vi "rsscope_core_global.vi"() -> ()   [LabVIEW 2018] (continued)
indicates the length of the data byte."}, {"Level"=4, "Class Only"=FALSE, "Identifier"="RSSCOPE_ATTR_CXPI_TRIGGER_DLC_CONDITION", "Descriptive Name"="CXPI Trigger DLC Condition", "Data Type"=0, "Command"="TRIG{Trigger}:CXPI:DLC:COND", "Access"=2, "Range Table"="rsscope_rngProtocolTriggerCondition", "Read Callback"="", "Write Callback"="", "Supported Models"="", "Instrument Options"="K76", "Flags"=0, "Help"="Set the condition for the DLC. You can define an exact value or a value range.\n\nAvailable Repeated Capabilities:\nTrigger: TrigA, TrigB, TrigR\r\n\nRemote-control command(s):\nTRIGger<m>:CXPI:DLC:CONDition"}, {"Level"=4, "Class Only"=FALSE, "Identifier"="RSSCOPE_ATTR_CXPI_TRIGGER_DLC_MIN", "Descriptive Name"="CXPI Trigger DLC Min", "Data Type"=2, "Command"="TRIG{Trigger}:CXPI:DLC:MIN", "Access"=2, "Range Table"="", "Read Callback"="", "Write Callback"="", "Supported Models"="", "Instrument Options"="K76", "Flags"=0, "Help"="Specifies a DLC pattern, or sets the start value of a pattern range.\n\nValid Values:\nBinary pattern string consisting of 1; 0; or X (any bit).\n\nAvailable Repeated Capabilities:\nTrigger: TrigA, TrigB, TrigR\r\n\nRemote-control command(s):\nTRIGger<m>:CXPI:DLC:MIN"}, {"Level"=4, "Class Only"=FALSE, "Identifier"="RSSCOPE_ATTR_CXPI_TRIGGER_DLC_MAX", "Descriptive Name"="CXPI Trigger DLC Max", "Data Type"=2, "Command"="TRIG{Trigger}:CXPI:DLC:MAX", "Access"=2, "Range Table"="", "Read Callback"="", "Write Callback"="", "Supported Models"="", "Instrument Options"="K76", "Flags"=0, "Help"="Sets the end value of a data type range for condition In Range or Out of Range. \n\nValid Values:\nBinary pattern string consisting of 1; 0; or X (any bit).\n\nAvailable Repeated Capabilities:\nTrigger: TrigA, TrigB, TrigR\r\n\nRemote-control command(s):\nTRIGger<m>:CXPI:DLC:MAX"}, {"Level"=3, "Class Only"=TRUE, "Identifier"="", "Descriptive Name"="DLC Extend", "Data Type"=0, "Command"="", "Access"=0, "Range Table"="", "Read Callback"="", "Write Callback"="", "Supported Models"="", "Instrument Options"="", "Flags"=0, "Help"="Sets the extension data length code, which indicates the length of the data byte of a long frame."}, {"Level"=4, "Class Only"=FALSE, "Identifier"="RSSCOPE_ATTR_CXPI_TRIGGER_DLC_EXTEND_CONDITION", "Descriptive Name"="CXPI Trigger DLC Extend Condition", "Data Type"=0, "Command"="TRIG{Trigger}:CXPI:DEXT:COND", "Access"=2, "Range Table"="rsscope_rngProtocolTriggerCondition", "Read Callback"="", "Write Callback"="", "Supported Models"="", "Instrument Options"="K76", "Flags"=0, "Help"="Set the condition for the DLC extend value. You can define an exact value or a value range.\n\nAvailable Repeated Capabilities:\nTrigger: TrigA, TrigB, TrigR\r\n\nRemote-control command(s):\nTRIGger<m>:CXPI:DEXTension:CONDition"}, {"Level"=4, "Class Only"=FALSE, "Identifier"="RSSCOPE_ATTR_CXPI_TRIGGER_DLC_EXTEND_MIN", "Descriptive Name"="CXPI Trigger DLC Extend Min", "Data Type"=2, "Command"="TRIG{Trigger}:CXPI:DEXT:MIN", "Access"=2, "Range Table"="", "Read Callback"="", "Write Callback"="", "Supported Models"="", "Instrument Options"="K76", "Flags"=0, "Help"="Specifies a data extension bit pattern, or sets the start value of a pattern range.\n\nValid Values:\nBinary pattern string consisting of 1; 0; or X (any bit).\n\nAvailable Repeated Capabilities:\nTrigger: TrigA, TrigB, TrigR\r\n\nRemote-control command(s):\nTRIGger<m>:CXPI:DEXTension:MIN"}, {"Level"=4, "Class Only"=FALSE, "Identifier"="RSSCOPE_ATTR_CXPI_TRIGGER_DLC_EXTEND_MAX", "Descriptive Name"="CXPI Trigger DLC Extend Max", "Data Type"=2, "Command"="TRIG{Trigger}:CXPI:DEXT:MAX", "Access"=2, "Range Table"="", "Read Callback"="", "Write Callback"="", "Supported Models"="", "Instrument Options"="K76", "Flags"=0, "Help"="Sets the end value of a DLC extend range for condition In Range or Out of Range. \n\nValid Values:\nBinary pattern string consisting of 1; 0; or X (any bit).\n\nAvailable Repeated Capabilities:\nTrigger: TrigA, TrigB, TrigR\r\n\nRemote-control command(s):\nTRIGger<m>:CXPI:DEXTension:MAX"}, {"Level"=3, "Class Only"=TRUE, "Identifier"="", "Descriptive Name"="Data", "Data Type"=0, "Command"="", "Access"=0, "Range Table"="", "Read Callback"="", "Write Callback"="", "Supported Models"="", "Instrument Options"="", "Flags"=0, "Help"="The data setup consists of the condition and one or two identifier pattern."}, {"Level"=4, "Class Only"=FALSE, "Identifier"="RSSCOPE_ATTR_CXPI_TRIGGER_DATA_CONDITION", "Descriptive Name"="CXPI Trigger Data Condition", "Data Type"=0, "Command"="TRIG{Trigger}:CXPI:DATA:DCON", "Access"=2, "Range Table"="rsscope_rngCXPIDataCondition", "Read Callback"="", "Write Callback"="", "Supported Models"="", "Instrument Options"="K76", "Flags"=0, "Help"="Sets the condition for the data pattern. You can define no value, an exact value or a value range.\n\nAvailable Repeated Capabilities:\nTrigger: TrigA, TrigB, TrigR\r\n\nRemote-control command(s):\nTRIGger<m>:CXPI:DATA:DCONdition"}, {"Level"=4, "Class Only"=FALSE, "Identifier"="RSSCOPE_ATTR_CXPI_TRIGGER_DATA_MIN", "Descriptive Name"="CXPI Trigger Data Min", "Data Type"=2, "Command"="TRIG{Trigger}:CXPI:DATA:DMIN", "Access"=2, "Range Table"="", "Read Callback"="", "Write Callback"="", "Supported Models"="", "Instrument Options"="K76", "Flags"=0, "Help"="Specifies a data bit pattern, or sets the start value of a pattern range.\n\nValid Values:\nBinary pattern string consisting of 1; 0; or X (any bit).\n\nAvailable Repeated Capabilities:\nTrigger: TrigA, TrigB, TrigR\r\n\nRemote-control command(s):\nTRIGger<m>:CXPI:DATA:DMIN"}, {"Level"=4, "Class Only"=FALSE, "Identifier"="RSSCOPE_ATTR_CXPI_TRIGGER_DATA_MAX", "Descriptive Name"="CXPI Trigger Data Max", "Data Type"=2, "Command"="TRIG{Trigger}:CXPI:DATA:DMAX", "Access"=2, "Range Table"="", "Read Callback"="", "Write Callback"="", "Supported Models"="", "Instrument Options"="K76", "Flags"=0, "Help"="Sets the end value of a data type range for condition In Range or Out of Range. \n\nValid Values:\nBinary pattern string consisting of 1; 0; or X (any bit).\n\nAvailable Repeated Capabilities:\nTrigger: TrigA, TrigB, TrigR\r\n\nRemote-control command(s):\nTRIGger<m>:CXPI:DATA:DMAX"}, {"Level"=3, "Class Only"=TRUE, "Identifier"="", "Descriptive Name"="Index", "Data Type"=0, "Command"="", "Access"=0, "Range Table"="", "Read Callback"="", "Write Callback"="", "Supported Models"="", "Instrument Options"="", "Flags"=0, "Help"="The data index setup consists of the condition and one or two index patterns."}, {"Level"=4, "Class Only"=FALSE, "Identifier"="RSSCOPE_ATTR_CXPI_TRIGGER_INDEX_CONDITION", "Descriptive Name"="CXPI Trigger Index Condition", "Data Type"=0, "Command"="TRIG{Trigger}:CXPI:DATA:ICON", "Access"=2, "Range Table"="rsscope_rngProtocolTriggerCondition", "Read Callback"="", "Write Callback"="", "Supported Models"="", "Instrument Options"="K76", "Flags"=0, "Help"="Set the condition for the data index value. You can define an exact value or a value range.\n\nAvailable Repeated Capabilities:\nTrigger: TrigA, TrigB, TrigR\r\n\nRemote-control command(s):\nTRIGger<m>:CXPI:DATA:ICONdition"}, {"Level"=4, "Class Only"=FALSE, "Identifier"="RSSCOPE_ATTR_CXPI_TRIGGER_INDEX_MIN", "Descriptive Name"="CXPI Trigger Index Min", "Data Type"=0, "Command"="TRIG{Trigger}:CXPI:DATA:IMIN", "Access"=2, "Range Table"="", "Read Callback"="", "Write Callback"="", "Supported Models"="", "Instrument Options"="K76", "Flags"=0, "Help"="Specifies a data index bit pattern, or sets the start value of a pattern range.\n\nAvailable Repeated Capabilities:\nTrigger: TrigA, TrigB, TrigR\r\n\nRemote-control command(s):\nTRIGger<m>:CXPI:DATA:IMIN"}, {"Level"=4, "Class Only"=FALSE, "Identifier"="RSSCOPE_ATTR_CXPI_TRIGGER_INDEX_MAX", "Descriptive Name"="CXPI Trigger Index Max", "Data Type"=0, "Command"="TRIG{Trigger}:CXPI:DATA:IMAX", "Access"=2, "Range Table"="", "Read Callback"="", "Write Callback"="", "Supported Models"="", "Instrument Options"="K76", "Flags"=0, "Help"="Sets the end value of a data index range for condition In Range or Out of Range.\n\nAvailable Repeated Capabilities:\nTrigger: TrigA, TrigB, TrigR\r\n\nRemote-control command(s):\nTRIGger<m>:CXPI:DATA:IMAX"}, {"Level"=3, "Class Only"=TRUE, "Identifier"="", "Descriptive Name"="Error", "Data Type"=0, "Command"="", "Access"=0, "Range Table"="", "Read Callback"="", "Write Callback"="", "Supported Models"="", "Instrument Options"="", "Flags"=0, "Help"="Trigger on selected error types."}, {"Level"=4, "Class Only"=FALSE, "Identifier"="RSSCOPE_ATTR_CXPI_TRIGGER_ERROR_CRC", "Descriptive Name"="CXPI Trigger Error CRC", "Data Type"=3, "Command"="TRIG{Trigger}:CXPI:ERR:CRC", "Access"=2, "Range Table"="", "Read Callback"="", "Write Callback"="", "Supported Models"="", "Instrument Options"="K76", "Flags"=0, "Help"="Triggers on a cyclic redundancy check error.\n\nAvailable Repeated Capabilities:\nTrigger: TrigA, TrigB, TrigR\r\n\nRemote-control command(s):\nTRIGger<m>:CXPI:ERRor:CRC"}, {"Level"=4, "Class Only"=FALSE, "Identifier"="RSSCOPE_ATTR_CXPI_TRIGGER_ERROR_DLC", "Descriptive Name"="CXPI Trigger Error DLC", "Data Type"=3, "Command"="TRIG{Trigger}:CXPI:ERR:DLC", "Access"=2, "Range Table"="", "Read Callback"="", "Write Callback"="", "Supported Models"="", "Instrument Options"="K76", "Flags"=0, "Help"="Triggers on a data length code (DLC) error.\n\nAvailable Repeated Capabilities:\nTrigger: TrigA, TrigB, TrigR\r\n\nRemote-control command(s):\nTRIGger<m>:CXPI:ERRor:DLC"}, {"Level"=4, "Class Only"=FALSE, "Identifier"="RSSCOPE_ATTR_CXPI_TRIGGER_ERROR_IBS", "Descriptive Name"="CXPI Trigger Error IBS", "Data Type"=3, "Command"="TRIG{Trigger}:CXPI:ERR:IBS", "Access"=2, "Range Table"="", "Read Callback"="", "Write Callback"="", "Supported Models"="", "Instrument Options"="K76", "Flags"=0, "Help"="Triggers on an inter-byte-space (IBS) error.\n\nAvailable Repeated Capabilities:\nTrigger: TrigA, TrigB, TrigR\r\n\nRemote-control command(s):\nTRIGger<m>:CXPI:ERRor:IBS"}, {"Level"=4, "Class Only"=FALSE, "Identifier"="RSSCOPE_ATTR_CXPI_TRIGGER_ERROR_IFS", "Descriptive Name"="CXPI Trigger Error IFS", "Data Type"=3, "Command"="TRIG{Trigger}:CXPI:ERR:IFS", "Access"=2, "Range Table"="", "Read Callback"="", "Write Callback"="", "Supported Models"="", "Instrument Options"="K76", "Flags"=0, "Help"="Triggers on an inter-frame-space (IFS) error.\n\nAvailable Repeated Capabilities:\nTrigger: TrigA, TrigB, TrigR\r\n\nRemote-control command(s):\nTRIGger<m>:CXPI:ERRor:IFS"}, {"Level"=4, "Class Only"=FALSE, "Identifier"="RSSCOPE_ATTR_CXPI_TRIGGER_ERROR_LENGTH", "Descriptive Name"="CXPI Trigger Error Length", "Data Type"=3, "Command"="TRIG{Trigger}:CXPI:ERR:LENG", "Access"=2, "Range Table"="", "Read Callback"="", "Write Callback"="", "Supported Models"="", "Instrument Options"="K76", "Flags"=0, "Help"="Triggers on a length error.\n\nAvailable Repeated Capabilities:\nTrigger: TrigA, TrigB, TrigR\r\n\nRemote-control command(s):\nTRIGger<m>:CXPI:ERRor:LENGth"}, {"Level"=4, "Class Only"=FALSE, "Identifier"="RSSCOPE_ATTR_CXPI_TRIGGER_ERROR_PARITY", "Descriptive Name"="CXPI Trigger Error Parity", "Data Type"=3, "Command"="TRIG{Trigger}:CXPI:ERR:PAR", "Access"=2, "Range Table"="", "Read Callback"="", "Write Callback"="", "Supported Models"="", "Instrument Options"="K76", "Flags"=0, "Help"="Triggers on a parity error indicating a transmission error.\n\nAvailable Repeated Capabilities:\nTrigger: TrigA, TrigB, TrigR\r\n\nRemote-control command(s):\nTRIGger<m>:CXPI:ERRor:PARity"}, {"Level"=4, "Class Only"=FALSE, "Identifier"="RSSCOPE_ATTR_CXPI_TRIGGER_ERROR_UART", "Descriptive Name"="CXPI Trigger Error UART", "Data Type"=3, "Command"="TRIG{Trigger}:CXPI:ERR:UART", "Access"=2, "Range Table"="", "Read Callback"="", "Write Callback"="", "Supported Models"="", "Instrument Options"="K76", "Flags"=0, "Help"="Triggers on an UART error.\n\nAvailable Repeated Capabilities:\nTrigger: TrigA, TrigB, TrigR\r\n\nRemote-control command(s):\nTRIGger<m>:CXPI:ERRor:UART"}, {"Level"=2, "Class Only"=TRUE, "Identifier"="", "Descriptive Name"="PCIe", "Data Type"=0, "Command"="", "Access"=0, "Range Table"="", "Read Callback"="", "Write Callback"="", "Supported Models"="", "Instrument Options"="", "Flags"=0, "Help"="Configures PCIe trigger."}, {"Level"=3, "Class Only"=FALSE, "Identifier"="RSSCOPE_ATTR_PCIE_TRIGGER_TYPE", "Descriptive Name"="PCIe Trigger Type", "Data Type"=0, "Command"="TRIG{Trigger}:PCIE:TYPE", "Access"=2, "Range Table"="RsScope_rngPCIeTriggerType", "Read Callback"="", "Write Callback"="", "Supported Models"="RTO|RTP", "Instrument Options"="K72", "Flags"=0, "Help"="Sets the trigger type for the PCI express analysis.\n\nAvailable Repeated Capabilities:\nTrigger: TrigA, TrigB, TrigR\r\n\nRemote-control command(s):\nTRIGger<m>:PCIE:TYPE"}, {"Level"=3, "Class Only"=FALSE, "Identifier"="RSSCOPE_ATTR_PCIE_TRIGGER_LEVEL", "Descriptive Name"="PCIe Trigger Level", "Data Type"=1, "Command"="TRIG{Trigger}:PCIE:TRGL", "Access"=2, "Range Table"="RsScope_rngPCIeTriggerLevel", "Read Callback"="", "Write Callback"="", "Supported Models"="", "Instrument Options"="", "Flags"=0, "Help"="Sets the trigger level for PCIe Gen 3.\n\nAvailable Repeated Capabilities:\nTrigger: TrigA, TrigB, TrigR\r\n\nRemote-control command(s):\nTRIGger<m>:PCIE:TRGLevel"}, {"Level"=3, "Class Only"=TRUE, "Identifier"="", "Descriptive Name"="TLP", "Data Type"=0, "Command"="", "Access"=0, "Range Table"="", "Read Callback"="", "Write Callback"="", "Supported Models"="", "Instrument Options"="", "Flags"=0, "Help"="Triggers on a transaction type."}, {"Level"=4, "Class Only"=FALSE, "Identifier"="RSSCOPE_ATTR_PCIE_TRIGGER_TLP", "Descriptive Name"="PCIe Trigger TLP", "Data Type"=0, "Command"="TRIG{Trigger}:PCIE:TLP:TYPE", "Access"=2, "Range Table"="RsScope_rngPCIeTLP", "Read Callback"="", "Write Callback"="", "Supported Models"="RTO|RTP", "Instrument Options"="K72", "Flags"=0, "Help"="Sets the transaction type to be triggered on for the transaction layer type trigger.\n\nAvailable Repeated Capabilities:\nTrigger: TrigA, TrigB, TrigR\r\n\nRemote-control command(s):\nTRIGger<m>:PCIE:TLP:TYPE"}, {"Level"=4, "Class Only"=FALSE, "Identifier"="RSSCOPE_ATTR_PCIE_TRIGGER_TLP_SEQUENCE_NUMBER", "Descriptive Name"="PCIe Trigger TLP Sequence Number", "Data Type"=2, "Command"="TRIG{Trigger}:PCIE:TLP:SNUM", "Access"=2, "Range Table"="", "Read Callback"="", "Write Callback"="", "Supported Models"="RTO|RTP", "Instrument Options"="K72", "Flags"=0, "Help"="Sets the sequence number to be triggered on for the transaction layer type trigger.\n\nAvailable Repeated Capabilities:\nTrigger: TrigA, TrigB, TrigR\r\n\nRemote-control command(s):\nTRIGger<m>:PCIE:TLP:SNUM"}, {"Level"=4, "Class Only"=FALSE, "Identifier"="RSSCOPE_ATTR_PCIE_TRIGGER_TLP_TC", "Descriptive Name"="PCIe Trigger TLP TC", "Data Type"=0, "Command"="TRIG{Trigger}:PCIE:TLP:TCHN", "Access"=2, "Range Table"="RsScope_rngPCIeTLPTC", "Read Callback"="", "Write Callback"="", "Supported Models"="RTO|RTP", "Instrument Options"="K72", "Flags"=0, "Help"="Sets the traffic class to be triggered on for the transaction layer type trigger.\n\nAvailable Repeated Capabilities:\nTrigger: TrigA, TrigB, TrigR\r\n\nRemote-control command(s):\nTRIGger<m>:PCIE:TLP:TCHN"}, {"Level"=4, "Class Only"=FALSE, "Identifier"="RSSCOPE_ATTR_PCIE_TRIGGER_TLP_ORDERING", "Descriptive Name"="PCIe Trigger TLP Ordering", "Data Type"=0, "Command"="TRIG{Trigger}:PCIE:TLP:ORDE", "Access"=2, "Range Table"="RsScope_rngPCIeTLPOrdering", "Read Callback"="", "Write Callback"="", "Supported Models"="RTO|RTP", "Instrument Options"="K72", "Flags"=0, "Help"="Sets the ordering type to be triggered on for the transaction layer type trigger.\n\nAvailable Repeated Capabilities:\nTrigger: TrigA, TrigB, TrigR\r\n\nRemote-control command(s):\nTRIGger<m>:PCIE:TLP:ORDE"}, {"Level"=4, "Class Only"=FALSE, "Identifier"="RSSCOPE_ATTR_PCIE_TRIGGER_TLP_SNOOP", "Descriptive Name"="PCIe Trigger TLP Snoop", "Data Type"=0, "Command"="TRIG{Trigger}:PCIE:TLP:SNOO", "Access"=2, "Range Table"="RsScope_rngPCIeTLPSnoop", "Read Callback"="", "Write Callback"="", "Supported Models"="RTO|RTP", "Instrument Options"="K72", "Flags"=0, "Help"="Triggers on a snoop state.\n\nAvailable Repeated Capabilities:\nTrigger: TrigA, TrigB, TrigR\r\n\nRemote-control command(s):\nTRIGger<m>:PCIE:TLP:SNOO"}, {"Level"=4, "Class Only"=FALSE, "Identifier"="RSSCOPE_ATTR_PCIE_TRIGGER_TLP_REQUESTER_ID", "Descriptive Name"="PCIe Trigger TLP Requester ID", "Data Type"=2, "Command"="TRIG{Trigger}:PCIE:TLP:REID", "Access"=2, "Range Table"="", "Read Callback"="", "Write Callback"="", "Supported Models"="RTO|RTP", "Instrument Options"="K72", "Flags"=0, "Help"="Sets the requester ID to be triggered on for the transaction layer type trigger.\n\nAvailable Repeated Capabilities:\nTrigger: TrigA, TrigB, TrigR\r\n\nRemote-control command(s):\nTRIGger<m>:PCIE:TLP:REID"}, {"Level"=4, "Class Only"=FALSE, "Identifier"="RSSCOPE_ATTR_PCIE_TRIGGER_TLP_DEVICE_ID", "Descriptive Name"="PCIe Trigger TLP Device ID", "Data Type"=2, "Command"="TRIG{Trigger}:PCIE:TLP:DEID", "Access"=2, "Range Table"="", "Read Callback"="", "Write Callback"="", "Supported Models"="RTO|RTP", "Instrument Options"="K72", "Flags"=0, "Help"="Sets the device ID to be triggered on for the transaction layer type trigger.\n\nAvailable Repeated Capabilities:\nTrigger: TrigA, TrigB, TrigR\r\n\nRemote-control command(s):\nTRIGger<m>:PCIE:TLP:DEID"}, {"Level"=4, "Class Only"=FALSE, "Identifier"="RSSCOPE_ATTR_PCIE_TRIGGER_TLP_READ_WRITE", "Descriptive Name"="PCIe Trigger TLP Read Write", "Data Type"=0, "Command"="TRIG{Trigger}:PCIE:TLP:MERW", "Access"=2, "Range Table"="RsScope_rngPCIeTLPReadWrite", "Read Callback"="", "Write Callback"="", "Supported Models"="RTO|RTP", "Instrument Options"="K72", "Flags"=0, "Help"="Sets the read/ write type to be triggered on for the transaction layer type trigger.\n\nAvailable Repeated Capabilities:\nTrigger: TrigA, TrigB, TrigR\r\n\nRemote-control command(s):\nTRIGger<m>:PCIE:TLP:MERW"}, {"Level"=4, "Class Only"=FALSE, "Identifier"="RSSCOPE_ATTR_PCIE_TRIGGER_TLP_ADDRESS_TYPE", "Descriptive Name"="PCIe Trigger TLP Address Type", "Data Type"=0, "Command"="TRIG{Trigger}:PCIE:TLP:ADRT", "Access"=2, "Range Table"="RsScope_rngPCIeTLPAddressType", "Read Callback"="", "Write Callback"="", "Supported Models"="RTO|RTP", "Instrument Options"="K72", "Flags"=0, "Help"="Sets the address type to be triggered on for the transaction layer type trigger.\n\nAvailable Repeated Capabilities:\nTrigger: TrigA, TrigB, TrigR\r\n\nRemote-control command(s):\nTRIGger<m>:PCIE:TLP:ADRT"}, {"Level"=4, "Class Only"=FALSE, "Identifier"="RSSCOPE_ATTR_PCIE_TRIGGER_TLP_TYPE", "Descriptive Name"="PCIe Trigger TLP Type", "Data Type"=0, "Command"="TRIG{Trigger}:PCIE:TLP:CFGT", "Access"=2, "Range Table"="RsScope_rngPCIeTLPType", "Read Callback"="", "Write Callback"="", "Supported Models"="RTO|RTP", "Instrument Options"="K72", "Flags"=0, "Help"="Triggers on a configuration type.\n\nAvailable Repeated Capabilities:\nTrigger: TrigA, TrigB, TrigR\r\n\nRemote-control command(s):\nTRIGger<m>:PCIE:TLP:CFGT"}, {"Level"=4, "Class Only"=FALSE, "Identifier"="RSSCOPE_ATTR_PCIE_TRIGGER_TLP_AT_TYPE", "Descriptive Name"="PCIe Trigger TLP AT Type", "Data Type"=0, "Command"="TRIG{Trigger}:PCIE:TLP:AT", "Access"=2, "Range Table"="RsScope_rngTriggerTLPATType", "Read Callback"="", "Write Callback"="", "Supported Models"="", "Instrument Options"="", "Flags"=0, "Help"="Sets the AT Type.\n\nAvailable Repeated Capabilities:\nTrigger: TrigA, TrigB, TrigR\r\n\nRemote-control command(s):\nTRIGger<m>:PCIE:TLP:AT"}, {"Level"=4, "Class Only"=FALSE, "Identifier"="RSSCOPE_ATTR_PCIE_TRIGGER_TLP_ROUTING", "Descriptive Name"="PCIe Trigger TLP Routing", "Data Type"=0, "Command"="TRIG{Trigger}:PCIE:TLP:MSGR", "Access"=2, "Range Table"="RsScope_rngPCIeTLPRouting", "Read Callback"="", "Write Callback"="", "Supported Models"="RTO|RTP", "Instrument Options"="K72", "Flags"=0, "Help"="Sets the message routing type to be triggered on for the transaction layer type trigger.\n\nAvailable Repeated Capabilities:\nTrigger: TrigA, TrigB, TrigR\r\n\nRemote-control command(s):\nTRIGger<m>:PCIE:TLP:MSGR"}, {"Level"=4, "Class Only"=FALSE, "Identifier"="RSSCOPE_ATTR_PCIE_TRIGGER_TLP_MESSAGE_CODE", "Descriptive Name"="PCIe Trigger TLP Message Code", "Data Type"=2, "Command"="TRIG{Trigger}:PCIE:TLP:MSGC", "Access"=2, "Range Table"="", "Read Callback"="", "Write Callback"="", "Supported Models"="RTO|RTP", "Instrument Options"="K72", "Flags"=0, "Help"="Sets the message code to be triggered on for the transaction layer type trigger.\n\nAvailable Repeated Capabilities:\nTrigger: TrigA, TrigB, TrigR\r\n\nRemote-control command(s):\nTRIGger<m>:PCIE:TLP:MSGC"}, {"Level"=4, "Class Only"=FALSE, "Identifier"="RSSCOPE_ATTR_PCIE_TRIGGER_TLP_STATUS", "Descriptive Name"="PCIe Trigger TLP Status", "Data Type"=0, "Command"="TRIG{Trigger}:PCIE:TLP:CPLS", "Access"=2, "Range Table"="RsScope_rngPCIeTLPStatus", "Read Callback"="", "Write Callback"="", "Supported Models"="RTO|RTP", "Instrument Options"="K72", "Flags"=0, "Help"="Sets the completion status to be triggered on for the transaction layer type trigger.\n\nAvailable Repeated Capabilities:\nTrigger: TrigA, TrigB, TrigR\r\n\nRemote-control command(s):\nTRIGger<m>:PCIE:TLP:CPLS"}, {"Level"=4, "Class Only"=FALSE, "Identifier"="RSSCOPE_ATTR_PCIE_TRIGGER_TLP_COMPLETER_ID", "Descriptive Name"="PCIe Trigger TLP Completer ID", "Data Type"=2, "Command"="TRIG{Trigger}:PCIE:TLP:CPID", "Access"=2, "Range Table"="", "Read Callback"="", "Write Callback"="", "Supported Models"="RTO|RTP", "Instrument Options"="K72", "Flags"=0, "Help"="Sets the completer ID to be triggered on for the transaction layer type trigger.\n\nAvailable Repeated Capabilities:\nTrigger: TrigA, TrigB, TrigR\r\n\nRemote-control command(s):\nTRIGger<m>:PCIE:TLP:CPID"}, {"Level"=3, "Class Only"=TRUE, "Identifier"="", "Descriptive Name"="DLLP", "Data Type"=0, "Command"="", "Access"=0, "Range Table"="", "Read Callback"="", "Write Callback"="", "Supported Models"="", "Instrument Options"="", "Flags"=0, "Help"="Configures data link layer trigger."}, {"Level"=4, "Class Only"=FALSE, "Identifier"="RSSCOPE_ATTR_PCIE_TRIGGER_DLLP", "Descriptive Name"="PCIe Trigger DLLP", "Data Type"=0, "Command"="TRIG{Trigger}:PCIE:DLLP:TYPE", "Access"=2, "Range Table"="RsScope_rngPCIeDLLP", "Read Callback"="", "Write Callback"="", "Supported Models"="RTO|RTP", "Instrument Options"="K72", "Flags"=0, "Help"="Sets the DLLP t type to be triggered on for the data link layer trigger.\n\nAvailable Repeated Capabilities:\nTrigger: TrigA, TrigB, TrigR\r\n\nRemote-control command(s):\nTRIGger<m>:PCIE:DLLP:TYPE"}, {"Level"=4, "Class Only"=FALSE, "Identifier"="RSSCOPE_ATTR_PCIE_TRIGGER_DLLP_MR_TYPE", "Descriptive Name"="PCIe Trigger DLLP MR Type", "Data Type"=0, "Command"="TRIG{Trigger}:PCIE:DLLP:MULT:TYPE", "Access"=2, "Range Table"="RsScope_rngPCIeDLLPMRType", "Read Callback"="", "Write Callback"="", "Supported Models"="RTO|RTP", "Instrument Options"="K72", "Flags"=0, "Help"="Sets the multi-root type for the data link layer to be triggered on.\n\nAvailable Repeated Capabilities:\nTrigger: TrigA, TrigB, TrigR\r\n\nRemote-control command(s):\nTRIGger<m>:PCIE:DLLP:MULT:TYPE"}, {"Level"=4, "Class Only"=FALSE, "Identifier"="RSSCOPE_ATTR_PCIE_TRIGGER_DLLP_MR_INIT_PHASE", "Descriptive Name"="PCIe Trigger DLLP MR Init Phase", "Data Type"=0, "Command"="TRIG{Trigger}:PCIE:DLLP:MULT:PHAS", "Access"=2, "Range Table"="RsScope_rngPCIeState", "Read Callback"="", "Write Callback"="", "Supported Models"="RTO|RTP", "Instrument Options"="K72", "Flags"=0, "Help"="Sets the phase state to be triggered on for the data link layer trigger.\n\nAvailable Repeated Capabilities:\nTrigger: TrigA, TrigB, TrigR\r\n\nRemote-control command(s):\nTRIGger<m>:PCIE:DLLP:MULT:PHAS"}, {"Level"=4, "Class Only"=FALSE, "Identifier"="RSSCOPE_ATTR_PCIE_TRIGGER_DLLP_MR_INIT_VH_FC", "Descriptive Name"="PCIe Trigger DLLP MR Init VH FC", "Data Type"=0, "Command"="TRIG{Trigger}:PCIE:DLLP:MULT:VHFC", "Access"=2, "Range Table"="RsScope_rngPCIeState", "Read Callback"="", "Write Callback"="", "Supported Models"="RTO|RTP", "Instrument Options"="K72", "Flags"=0, "Help"="Sets the virtual hierarchies flow control presence state to be triggered on for the data link layer trigger.\n\nAvailable Repeated Capabilities:\nTrigger: TrigA, TrigB, TrigR\r\n\nRemote-control command(s):\nTRIGger<m>:PCIE:DLLP:MULT:VHFC"}, {"Level"=4, "Class Only"=FALSE, "Identifier"="RSSCOPE_ATTR_PCIE_TRIGGER_DLLP_MR_INIT_MIXED_TYPE", "Descriptive Name"="PCIe Trigger DLLP MR Init Mixed Type", "Data Type"=0, "Command"="TRIG{Trigger}:PCIE:DLLP:MULT:MIXT", "Access"=2, "Range Table"="RsScope_rngPCIeState", "Read Callback"="", "Write Callback"="", "Supported Models"="RTO|RTP", "Instrument Options"="K72", "Flags"=0, "Help"="Sets the mixed type presence state to be triggered on for the data link layer trigger.\n\nAvailable Repeated Capabilities:\nTrigger: TrigA, TrigB, TrigR\r\n\nRemote-control command(s):\nTRIGger<m>:PCIE:DLLP:MULT:MIXT"}, {"Level"=4, "Class Only"=FALSE, "Identifier"="RSSCOPE_ATTR_PCIE_TRIGGER_DLLP_MR_INIT_AUTHORIZED", "Descriptive Name"="PCIe Trigger DLLP MR Init Authorized", "Data Type"=0, "Command"="TRIG{Trigger}:PCIE:DLLP:MULT:AUTH", "Access"=2, "Range Table"="RsScope_rngPCIeState", "Read Callback"="", "Write Callback"="", "Supported Models"="RTO|RTP", "Instrument Options"="K72", "Flags"=0, "Help"="Sets the authorized presence state to be triggered on for the data link layer trigger.\n\nAvailable Repeated Capabilities:\nTrigger: TrigA, TrigB, TrigR\r\n\nRemote-control command(s):\nTRIGger<m>:PCIE:DLLP:MULT:AUTH"}, {"Level"=4, "Class Only"=FALSE, "Identifier"="RSSCOPE_ATTR_PCIE_TRIGGER_DLLP_MR_INIT_DEVICE_PORT_TYPE", "Descriptive Name"="PCIe Trigger DLLP MR Init Device Port Type", "Data Type"=0, "Command"="TRIG{Trigger}:PCIE:DLLP:MULT:DVPT", "Access"=2, "Range Table"="RsScope_rngPCIeDevicePortType", "Read Callback"="", "Write Callback"="", "Supported Models"="RTO|RTP", "Instrument Options"="K72", "Flags"=0, "Help"="Sets the device/port type to be triggered on for the data link layer trigger.\n\nAvailable Repeated Capabilities:\nTrigger: TrigA, TrigB, TrigR\r\n\nRemote-control command(s):\nTRIGger<m>:PCIE:DLLP:MULT:DVPT"}, {"Level"=4, "Class Only"=FALSE, "Identifier"="RSSCOPE_ATTR_PCIE_TRIGGER_DLLP_MR_VL_NUMBER", "Descriptive Name"="PCIe Trigger DLLP MR VL Number", "Data Type"=0, "Command"="TRIG{Trigger}:PCIE:DLLP:MULT:VLNR", "Access"=2, "Range Table"="RsScope_rngPCIeVLNumber", "Read Callback"="", "Write Callback"="", "Supported Models"="RTO|RTP", "Instrument Options"="K72", "Flags"=0, "Help"="Sets the virtual link (VL) number to be triggered on for the data link layer trigger.\n\nAvailable Repeated Capabilities:\nTrigger: TrigA, TrigB, TrigR\r\n\nRemote-control command(s):\nTRIGger<m>:PCIE:DLLP:MULT:VLNR"}, {"Level"=4, "Class Only"=FALSE, "Identifier"="RSSCOPE_ATTR_PCIE_TRIGGER_DLLP_MR_VH_ABSENT", "Descriptive Name"="PCIe Trigger DLLP MR VH Absent", "Data Type"=0, "Command"="TRIG{Trigger}:PCIE:DLLP:MULT:HABS", "Access"=2, "Range Table"="RsScope_rngPCIeState", "Read Callback"="", "Write Callback"="", "Supported Models"="RTO|RTP", "Instrument Options"="K72", "Flags"=0, "Help"="Sets the state of the absent virtual hieararchies (VH) to be triggered on for the data link layer trigger.\n\nAvailable Repeated Capabilities:\nTrigger: TrigA, TrigB, TrigR\r\n\nRemote-control command(s):\nTRIGger<m>:PCIE:DLLP:MULT:HABS"}, {"Level"=4, "Class Only"=FALSE, "Identifier"="RSSCOPE_ATTR_PCIE_TRIGGER_DLLP_MR_TLP_TYPE", "Descriptive Name"="PCIe Trigger DLLP MR TLP Type", "Data Type"=0, "Command"="TRIG{Trigger}:PCIE:DLLP:MULT:TLPT", "Access"=2, "Range Table"="RsScope_rngPCIeDLLPMRTLPType", "Read Callback"="", "Write Callback"="", "Supported Models"="RTO|RTP", "Instrument Options"="K72", "Flags"=0, "Help"="Sets the multi-root type to be triggered on for the data link layer trigger.\n\nAvailable Repeated Capabilities:\nTrigger: TrigA, TrigB, TrigR\r\n\nRemote-control command(s):\nTRIGger<m>:PCIE:DLLP:MULT:TLPT"}, {"Level"=4, "Class Only"=FALSE, "Identifier"="RSSCOPE_ATTR_PCIE_TRIGGER_DLLP_MR_CREDIT_TYPE", "Descriptive Name"="PCIe Trigger DLLP MR Credit Type", "Data Type"=0, "Command"="TRIG{Trigger}:PCIE:DLLP:MULT:CRET", "Access"=2, "Range Table"="RsScope_rngPCIeDLLPMRCreditType", "Read Callback"="", "Write Callback"="", "Supported Models"="RTO|RTP", "Instrument Options"="", "Flags"=0, "Help"="Sets the credit type to be triggered on for the multi-root data link layer trigger.\n\nAvailable Repeated Capabilities:\nTrigger: TrigA, TrigB, TrigR\r\n\nRemote-control command(s):\nTRIGger<m>:PCIE:DLLP:MULT:CRET"}, {"Level"=4, "Class Only"=FALSE, "Identifier"="RSSCOPE_ATTR_PCIE_TRIGGER_DLLP_MR_A", "Descriptive Name"="PCIe Trigger DLLP MR A", "Data Type"=0, "Command"="TRIG{Trigger}:PCIE:DLLP:MULT:RESA", "Access"=2, "Range Table"="RsScope_rngPCIeTriggerDLLPMRA", "Read Callback"="", "Write Callback"="", "Supported Models"="RTO|RTP", "Instrument Options"="K72", "Flags"=0, "Help"="Sets the on the value of the A bit to be triggered on for the data link layer trigger.\n\nAvailable Repeated Capabilities:\nTrigger: TrigA, TrigB, TrigR\r\n\nRemote-control command(s):\nTRIGger<m>:PCIE:DLLP:MULT:RESA"}, {"Level"=4, "Class Only"=FALSE, "Identifier"="RSSCOPE_ATTR_PCIE_TRIGGER_DLLP_MR_VH_GROUP", "Descriptive Name"="PCIe Trigger DLLP MR VH Group", "Data Type"=0, "Command"="TRIG{Trigger}:PCIE:DLLP:MULT:VHGR", "Access"=2, "Range Table"="RsScope_rngPCIeDLLPVHGroup", "Read Callback"="", "Write Callback"="", "Supported Models"="RTO|RTP", "Instrument Options"="K72", "Flags"=0, "Help"="Sets the virtual hierarchies group to be triggered on for the data link layer trigger.\n\nAvailable Repeated Capabilities:\nTrigger: TrigA, TrigB, TrigR\r\n\nRemote-control command(s):\nTRIGger<m>:PCIE:DLLP:MULT:VHGR"}, {"Level"=4, "Class Only"=FALSE, "Identifier"="RSSCOPE_ATTR_PCIE_TRIGGER_DLLP_SEQUENCE", "Descriptive Name"="PCIe Trigger DLLP Sequence", "Data Type"=2, "Command"="TRIG{Trigger}:PCIE:DLLP:SEQ", "Access"=2, "Range Table"="", "Read Callback"="", "Write Callback"="", "Supported Models"="RTO|RTP", "Instrument Options"="K72", "Flags"=0, "Help"="Sets the sequence field, indicating what TLPs are affected by the ACK/NAK, to be triggered on for the data link layer trigger.\n\nAvailable Repeated Capabilities:\nTrigger: TrigA, TrigB, TrigR\r\n\nRemote-control command(s):\nTRIGger<m>:PCIE:DLLP:SEQ"}, {"Level"=4, "Class Only"=FALSE, "Identifier"="RSSCOPE_ATTR_PCIE_TRIGGER_DLLP_FC_CREDIT_TYPE", "Descriptive Name"="PCIe Trigger DLLP FC Credit Type", "Data Type"=0, "Command"="TRIG{Trigger}:PCIE:DLLP:FCTL:CRET", "Access"=2, "Range Table"="RsScope_rngPCIeDLLPFCCreditType", "Read Callback"="", "Write Callback"="", "Supported Models"="RTO|RTP", "Instrument Options"="K72", "Flags"=0, "Help"="Sets credit type value to be triggered on for the data link layer trigger.\n\nAvailable Repeated Capabilities:\nTrigger: TrigA, TrigB, TrigR\r\n\nRemote-control command(s):\nTRIGger<m>:PCIE:DLLP:FCTL:CRET"}, {"Level"=4, "Class Only"=FALSE, "Identifier"="RSSCOPE_ATTR_PCIE_TRIGGER_DLLP_FC_VC_ID", "Descriptive Name"="PCIe Trigger DLLP FC VC ID", "Data Type"=0, "Command"="TRIG{Trigger}:PCIE:DLLP:FCTL:VCID", "Access"=2, "Range Table"="RsScope_rngPCIeDLLPVCID", "Read Callback"="", "Write Callback"="", "Supported Models"="RTO|RTP", "Instrument Options"="K72", "Flags"=0, "Help"="Sets the virtual channel ID to be triggered on for the data link layer trigger.\n\nAvailable Repeated Capabilities:\nTrigger: TrigA, TrigB, TrigR\r\n\nRemote-control command(s):\nTRIGger<m>:PCIE:DLLP:FCTL:VCID"}, {"Level"=4, "Class Only"=FALSE, "Identifier"="RSSCOPE_ATTR_PCIE_TRIGGER_DLLP_PM_TYPE", "Descriptive Name"="PCIe Trigger DLLP PM Type", "Data Type"=0, "Command"="TRIG{Trigger}:PCIE:DLLP:POWM", "Access"=2, "Range Table"="RsScope_rngPCIeDLLPPMType", "Read Callback"="", "Write Callback"="", "Supported Models"="RTO|RTP", "Instrument Options"="K72", "Flags"=0, "Help"="Sets the power management type to be triggered on for the data link layer trigger.\n\nAvailable Repeated Capabilities:\nTrigger: TrigA, TrigB, TrigR\r\n\nRemote-control command(s):\nTRIGger<m>:PCIE:DLLP:POWM"}, {"Level"=4, "Class Only"=FALSE, "Identifier"="RSSCOPE_ATTR_PCIE_TRIGGER_DLLP_VENDOR_PATTERN", "Descriptive Name"="PCIe Trigger DLLP Vendor Pattern", "Data Type"=2, "Command"="TRIG{Trigger}:PCIE:DLLP:VPAT", "Access"=2, "Range Table"="", "Read Callback"="", "Write Callback"="", "Supported Models"="RTO|RTP", "Instrument Options"="K72", "Flags"=0, "Help"="Sets the vendor pattern to be triggered on for the data link layer trigger.\n\nAvailable Repeated Capabilities:\nTrigger: TrigA, TrigB, TrigR\r\n\nRemote-control command(s):\nTRIGger<m>:PCIE:DLLP:VPAT"}, {"Level"=3, "Class Only"=TRUE, "Identifier"="", "Descriptive Name"="Ordered Sets", "Data Type"=0, "Command"="", "Access"=0, "Range Table"="", "Read Callback"="", "Write Callback"="", "Supported Models"="", "Instrument Options"="", "Flags"=0, "Help"="Configures the trigger on a defined ordered set."}, {"Level"=4, "Class Only"=FALSE, "Identifier"="RSSCOPE_ATTR_PCIE_TRIGGER_OSET_TYPE", "Descriptive Name"="PCIe Trigger OSET Type", "Data Type"=0, "Command"="TRIG{Trigger}:PCIE:OSET:TYPE", "Access"=2, "Range Table"="RsScope_rngPCIeOSETType", "Read Callback"="", "Write Callback"="", "Supported Models"="RTO|RTP", "Instrument Options"="K72", "Flags"=0, "Help"="Sets the ordered set to be triggered on.\n\nAvailable Repeated Capabilities:\nTrigger: TrigA, TrigB, TrigR\r\n\nRemote-control command(s):\nTRIGger<m>:PCIE:OSET:TYPE"}, {"Level"=3, "Class Only"=TRUE, "Identifier"="", "Descriptive Name"="Error Condition", "Data Type"=0, "Command"="", "Access"=0, "Range Table"="", "Read Callback"="", "Write Callback"="", "Supported Models"="", "Instrument Options"="", "Flags"=0, "Help"="Triggers on enabled error condition."}, {"Level"=4, "Class Only"=FALSE, "Identifier"="RSSCOPE_ATTR_PCIE_TRIGGER_ERRC_CRC16", "Descriptive Name"="PCIe Trigger ERRC CRC16 Error", "Data Type"=3, "Command"="TRIG{Trigger}:PCIE:ERRC:CRC", "Access"=2, "Range Table"="", "Read Callback"="", "Write Callback"="", "Supported Models"="RTO|RTP", "Instrument Options"="K72", "Flags"=0, "Help"="Enables triggering on 16-bit cyclic redundancy check (CRC) errors.\n\nAvailable Repeated Capabilities:\nTrigger: TrigA, TrigB, TrigR\r\n\nRemote-control command(s):\nTRIGger<m>:PCIE:ERRC:CRC"}, {"Level"=4, "Class Only"=FALSE, "Identifier"="RSSCOPE_ATTR_PCIE_TRIGGER_ERRC_LCRC", "Descriptive Name"="PCIe Trigger ERRC LCRC Error", "Data Type"=3, "Command"="TRIG{Trigger}:PCIE:ERRC:LCRC", "Access"=2, "Range Table"="", "Read Callback"="", "Write Callback"="", "Supported Models"="RTO|RTP", "Instrument Options"="K72", "Flags"=0, "Help"="Enables triggering on link cyclic redundancy check (LCRC) errors.\n\nAvailable Repeated Capabilities:\nTrigger: TrigA, TrigB, TrigR\r\n\nRemote-control command(s):\nTRIGger<m>:PCIE:ERRC:LCRC"}, {"Level"=4, "Class Only"=FALSE, "Identifier"="RSSCOPE_ATTR_PCIE_TRIGGER_ERRC_ECRC", "Descriptive Name"="PCIe Trigger ERRC ECRC Error", "Data Type"=3, "Command"="TRIG{Trigger}:PCIE:ERRC:ECRC", "Access"=2, "Range Table"="", "Read Callback"="", "Write Callback"="", "Supported Models"="RTO|RTP", "Instrument Options"="K72", "Flags"=0, "Help"="Enables triggering on end-to-end cyclic redundancy checksum (ECRC) errors.\n\nAvailable Repeated Capabilities:\nTrigger: TrigA, TrigB, TrigR\r\n\nRemote-control command(s):\nTRIGger<m>:PCIE:ERRC:ECRC"}, {"Level"=4, "Class Only"=FALSE, "Identifier"="RSSCOPE_ATTR_PCIE_TRIGGER_ERRC_INVALID_SYMBOL", "Descriptive Name"="PCIe Trigger ERRC Invalid Symbol", "Data Type"=3, "Command"="TRIG{Trigger}:PCIE:ERRC:INVP", "Access"=2, "Range Table"="", "Read Callback"="", "Write Callback"="", "Supported Models"="RTO|RTP", "Instrument Options"="K72", "Flags"=0, "Help"="Enables triggering on invalid symbol errors.\n\nAvailable Repeated Capabilities:\nTrigger: TrigA, TrigB, TrigR\r\n\nRemote-control command(s):\nTRIGger<m>:PCIE:ERRC:INVP"}, {"Level"=4, "Class Only"=FALSE, "Identifier"="RSSCOPE_ATTR_PCIE_TRIGGER_ERRC_DISP", "Descriptive Name"="PCIe Trigger ERRC Disparity Error", "Data Type"=3, "Command"="TRIG{Trigger}:PCIE:ERRC:DISP", "Access"=2, "Range Table"="", "Read Callback"="", "Write Callback"="", "Supported Models"="RTO|RTP", "Instrument Options"="K72", "Flags"=0, "Help"="Enables triggering on disparity errors.\n\nAvailable Repeated Capabilities:\nTrigger: TrigA, TrigB, TrigR\r\n\nRemote-control command(s):\nTRIGger<m>:PCIE:ERRC:DISP"}, {"Level"=4, "Class Only"=FALSE, "Identifier"="RSSCOPE_ATTR_PCIE_TRIGGER_ERRC_LENGTH", "Descriptive Name"="PCIe Trigger ERRC Length", "Data Type"=3, "Command"="TRIG{Trigger}:PCIE:ERRC:LENG", "Access"=2, "Range Table"="", "Read Callback"="", "Write Callback"="", "Supported Models"="RTO|RTP", "Instrument Options"="K72", "Flags"=0, "Help"="Enables triggering on a length error, for frames that do not have the specified length or data.\n\nAvailable Repeated Capabilities:\nTrigger: TrigA, TrigB, TrigR\r\n\nRemote-control command(s):\nTRIGger<m>:PCIE:ERRC:LENGth"}, {"Level"=4, "Class Only"=FALSE, "Identifier"="RSSCOPE_ATTR_PCIE_TRIGGER_ERRC_MALFORM_ERROR", "Descriptive Name"="PCIe Trigger ERRC Malform Error", "Data Type"=3, "Command"="TRIG{Trigger}:PCIE:ERRC:MALF", "Access"=2, "Range Table"="", "Read Callback"="", "Write Callback"="", "Supported Models"="RTO|RTP", "Instrument Options"="K72", "Flags"=0, "Help"="Enables triggering on a malformed TLP: a TLP that violates specific TLP formation rules that are defined in the specification.\n\nAvailable Repeated Capabilities:\nTrigger: TrigA, TrigB, TrigR\r\n\nRemote-control command(s):\nTRIGger<m>:PCIE:ERRC:MALFormed"}, {"Level"=4, "Class Only"=FALSE, "Identifier"="RSSCOPE_ATTR_PCIE_TRIGGER_ERRC_MAX_END_PREFIX", "Descriptive Name"="PCIe Trigger ERRC Max End Prefix", "Data Type"=3, "Command"="TRIG{Trigger}:PCIE:ERRC:MXPF", "Access"=2, "Range Table"="", "Read Callback"="", "Write Callback"="", "Supported Models"="RTO|RTP", "Instrument Options"="K72", "Flags"=0, "Help"="Enables triggering on an end-end prefix error. The maximum number of permitted end-end TLP prefixes is 4.\n\nAvailable Repeated Capabilities:\nTrigger: TrigA, TrigB, TrigR\r\n\nRemote-control command(s):\nTRIGger<m>:PCIE:ERRC:MXPFix"}, {"Level"=4, "Class Only"=FALSE, "Identifier"="RSSCOPE_ATTR_PCIE_TRIGGER_ERRC_PREFIX_ORDER_ERROR", "Descriptive Name"="PCIe Trigger ERRC Prefix Order Error", "Data Type"=3, "Command"="TRIG{Trigger}:PCIE:ERRC:PFOR", "Access"=2, "Range Table"="", "Read Callback"="", "Write Callback"="", "Supported Models"="RTO|RTP", "Instrument Options"="K72", "Flags"=0, "Help"="Enables triggering on a wrong prefix order.\n\nAvailable Repeated Capabilities:\nTrigger: TrigA, TrigB, TrigR\r\n\nRemote-control command(s):\nTRIGger<m>:PCIE:ERRC:PFORder"}, {"Level"=4, "Class Only"=FALSE, "Identifier"="RSSCOPE_ATTR_PCIE_TRIGGER_ERRC_SYNC_BIT", "Descriptive Name"="PCIe Trigger ERRC Sync Bit", "Data Type"=3, "Command"="TRIG{Trigger}:PCIE:ERRC:SYCB", "Access"=2, "Range Table"="", "Read Callback"="", "Write Callback"="", "Supported Models"="RTO|RTP", "Instrument Options"="K72", "Flags"=0, "Help"="Enables triggering on a sync bit.\n\nAvailable Repeated Capabilities:\nTrigger: TrigA, TrigB, TrigR\r\n\nRemote-control command(s):\nTRIGger<m>:PCIE:ERRC:SYCBit"}, {"Level"=4, "Class Only"=FALSE, "Identifier"="RSSCOPE_ATTR_PCIE_TRIGGER_ERRC_VALUE_OUT_OF_RANGE", "Descriptive Name"="PCIe Trigger ERRC Value Out Of Range", "Data Type"=3, "Command"="TRIG{Trigger}:PCIE:ERRC:VOOR", "Access"=2, "Range Table"="", "Read Callback"="", "Write Callback"="", "Supported Models"="RTO|RTP", "Instrument Options"="K72", "Flags"=0, "Help"="Ennables triggering, if a value of a field is out of the range defined by the PCIe standard.\n\nAvailable Repeated Capabilities:\nTrigger: TrigA, TrigB, TrigR\r\n\nRemote-control command(s):\nTRIGger<m>:PCIE:ERRC:VOORange"}, {"Level"=4, "Class Only"=FALSE, "Identifier"="RSSCOPE_ATTR_PCIE_TRIGGER_ERRC_UNKNOWN_PACKET", "Descriptive 
